vi "Configure Math (Advanced).vi"(7 "VAR2 (0)":dbl, 8 "error in (no error)":errorcluster, 9 "VAR1 (0)":dbl, 10 "Function (CH1+CH2)":string="CH1+CH2", 11 "VISA resource name":refnum<visa-resource-name>) -> (0 "error out":errorcluster, 3 "VISA resource name out":refnum<visa-resource-name>)   [LabVIEW 2009, in "Tektronix DPO MSO 2000 4000 Series.lvlib"]
doc: "Configures a math channel using a mathematical expression.\n\n<B>Note:</B>\n\nThis VI is invalid for DPO2K and MSO2K series."
uses:
  <instrlib>/Tektronix DPO MSO 2000 4000 Series/Tektronix DPO MSO 2000 4000 Series.lvlib
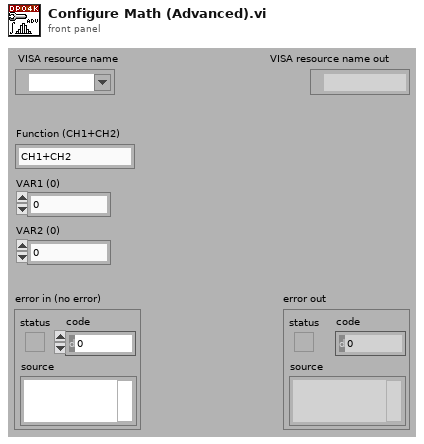
[diagram p1: front panel]
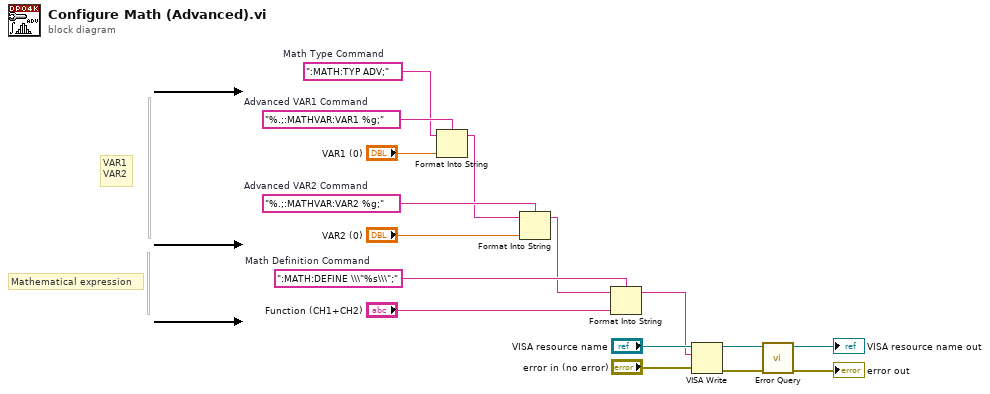
[diagram p0: block diagram]
diagram:
  w12 = ":MATH:DEFINE \\\"%s\\\";"  # Math Definition Command
  w13 = "%.;:MATHVAR:VAR2 %g;"  # Advanced VAR2 Command
  w15 = "%.;:MATHVAR:VAR1 %g;"  # Advanced VAR1 Command
  w8 = ":MATH:TYP ADV;"  # Math Type Command
  # "Mathematical expression"
  # "VAR1\nVAR2"
  n1 = Format Into String(format string=w15, initial string=w8, "VAR1 (0)") -> (resulting string=w7:string)  [unwired: 1 in, 1 out]
  n2 = Format Into String(format string=w13, initial string=w7, "VAR2 (0)") -> (resulting string=w6:string)  [unwired: 1 in, 1 out]
  n3 = Format Into String(format string=w12, initial string=w6, "Function (CH1+CH2)") -> (resulting string=w5:string)  [unwired: 1 in, 1 out]
  n4 = VISA Write(VISA resource name="VISA resource name", write buffer=w5, error in (no error)="error in (no error)") -> (VISA resource name out=w4:refnum<visa-resource-name>, error out=w3:errorcluster)  [unwired: 1 out]
  n5 = call <instrlib>:"Error Query.vi"("error in (no error)"=w3, "VISA resource name"=w4) -> ("error out"=→"error out":errorcluster, "VISA resource name out"=→"VISA resource name out":refnum<visa-resource-name>)  [unwired: 6 in, 2 out]
